vi "configure.vi"(8 "error in (no error)":errorcluster, 11 "DAQmxAnalogOut in":refnum<class "AnalogOutDL101207DAQmx.lvclass">) -> (0 "error out":errorcluster, 3 "DAQmxAnalogOut out":refnum<class "AnalogOutDL101207DAQmx.lvclass">)   [LabVIEW 2010, in "AnalogOutDL101207DAQmx.lvclass"]
doc: "The dynamic dispatch version of this VI loads and displays the configuration file associated with the plug-in object. The user modify and save the configuration data."
uses:
  AnalogOutDL101207DAQmx.lvclass
  AnalogOutDL101207DAQmx.lvclass/AnalogOutDL101207DAQmx.ctl
  common/classes/ErrorController/ErrorController/class_data.vi
  common/classes/GenericComponent/GenericComponent/GenericComponent.lvclass
  common/classes/ErrorController/ErrorController/ErrorController.lvclass
panel:
  out "Configuration":string
  in  "default voltage":dbl[unit]
  in  "cancel button":bool
  in  "save button":bool
  in  "maximum voltage":dbl[unit]
  in  "minimum voltage":dbl[unit]
  in  "DAQmx Physical Channel":tag
  # "Configure DAQmxAnalogOut"
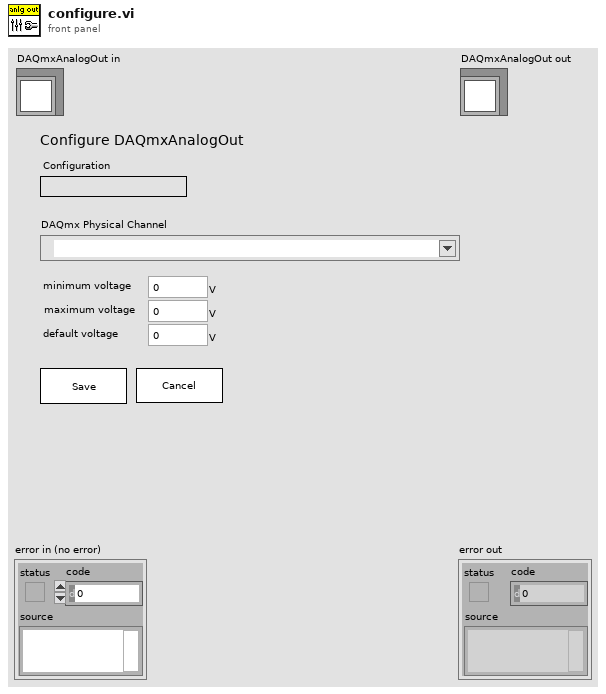
[diagram p1: front panel]
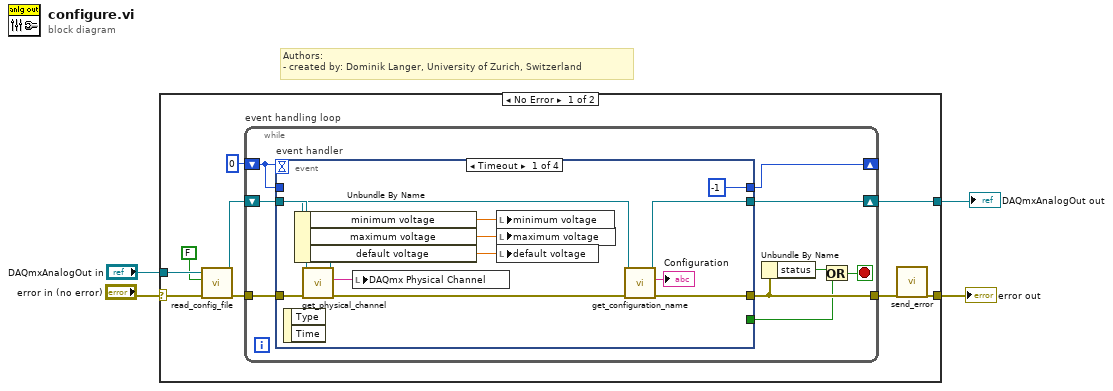
[diagram p0: block diagram]
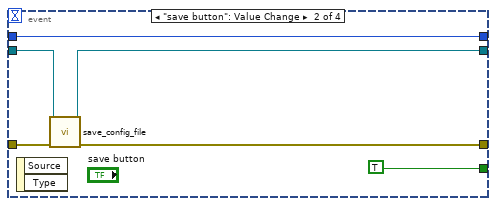
[diagram p2: hidden frame]
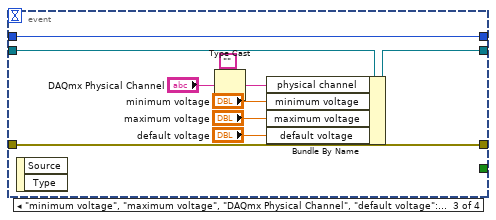
[diagram p3: hidden frame]
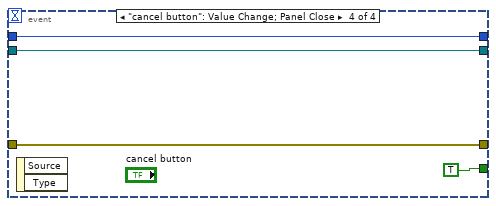
[diagram p4: hidden frame]
diagram:
  # "Authors: \n- created by: Dominik Langer, University of Zurich, Switzerland"
  n1 = case shown="No Error" "error in (no error)" {
    selector: "error in (no error)" -> [w11 w55]
    tunnel: [w13 w56] -> w2
    tunnel: "DAQmxAnalogOut in" -> [w9 w56]
    tunnel: [w6 w55] -> w1
    frame No Error {
      n2 = call-dynamic "read_config_file.vi"("error in (no error)"=w11, "force load?"=FALSE, "GenericPlugin in"=w9) -> ("error out"=w10:errorcluster, "GenericPlugin out"=w8:refnum<class "AnalogOutDL101207DAQmx.lvclass">)  [unwired: 7 out]
      n3 = while "event handling loop" {
        shift-right: [w20] -> w13
        shift-left: w8 -> [w21]
        shift-right: [w18] -> _
        shift-left: 0 -> [w19]
        tunnel: w10 -> [w22]
        tunnel: [w17] -> w5
        stop <- w14 stop-if-true
        n4 = event "event handler" shown="[0] Timeout" {
          selector: _ -> [_ _ _ _]
          dyn-events: _ -> [_ _ _ _]
          timeout: w19 -> [_ _ _ _]
          tunnel: w22 -> [w31 w38 w50 w54]
          tunnel: [w26 w36 w50 w54] -> w17
          tunnel: [w24 w37 w47 w53] -> w20
          tunnel: w21 -> [w29 w35 w48 w53]
          tunnel: [-1 w40 w49 w52] -> w18
          tunnel: w19 -> [_ w40 w49 w52]
          tunnel: [_ TRUE _ TRUE] -> w15
          event Timeout {
            n5 = event-data() -> ()  [unwired: 3 out]
            n6 = call-dynamic "get_physical_channel.vi"("error in (no error)"=w31, "DAQmxAnalogOut in"=w29) -> ("error out"=w27:errorcluster, "DAQmx Physical Channel"=w30:tag, "DAQmxAnalogOut out"=w25:refnum<class "AnalogOutDL101207DAQmx.lvclass">)  [unwired: 7 in]
            n7 = Unbundle By Name(w25) -> ("minimum voltage"=w33:dbl[unit], "maximum voltage"=w32:dbl[unit], "default voltage"=w28:dbl[unit])
            n8 = local write "DAQmx Physical Channel"(w30) -> ()
            n9 = local write "minimum voltage"(w33) -> ()
            n10 = local write "maximum voltage"(w32) -> ()
            n11 = local write "default voltage"(w28) -> ()
            n12 = call "get_configuration_name.vi"("error in (no error)"=w27, "GenericPlugin.lvclass in"=w25) -> ("error out"=w26:errorcluster, "configuration name"=→"Configuration":string, "GenericPlugin.lvclass out"=w24:refnum<class "AnalogOutDL101207DAQmx.lvclass">)  [unwired: 7 in]
          }
          event "save button": Value Change {
            n13 = event-data() -> ()  [unwired: 3 out]
            n14 = call-dynamic "save_config_file.vi"("error in (no error)"=w38, "GenericPlugin in"=w35) -> ("error out"=w36:errorcluster, "GenericPlugin out"=w37:refnum<class "AnalogOutDL101207DAQmx.lvclass">)  [unwired: 1 in, 7 out]
          }
          event "minimum voltage", "maximum voltage", "DAQmx Physical Channel", "default voltage": Value Change {
            n15 = event-data() -> ()  [unwired: 3 out]
            n16 = Type Cast(type="", x="DAQmx Physical Channel") -> (*(type *) &x=w42:string)
            n17 = Bundle By Name(cluster=w48, "physical channel"=w42, "minimum voltage"="minimum voltage", "maximum voltage"="maximum voltage", "default voltage"="default voltage") -> (w47:refnum<class "AnalogOutDL101207DAQmx.lvclass">)
          }
          event "cancel button": Value Change; Panel Close {
            n18 = event-data() -> ()  [unwired: 3 out]
          }
        }
        n19 = Unbundle By Name(w17) -> ("status"=w16:bool)
        n20 = Or(x=w16, y=w15) -> (x .or. y?=w14:bool)
      }
      n21 = call "send_error.vi"("error in (no error)"=w5) -> ("error out"=w6:errorcluster)  [unwired: 10 in]
    }
    frame Error {
    }
  }
  "error out" <- w1
  "DAQmxAnalogOut out" <- w2
